vi "SA Initialize - TOI.vi"(8 "error in":errorcluster, 11 "RFmx Settings":T1 {"Attenuation"."Attenuation"."s2p File"."RFmx S-Parameters Orientation" items=["Port1 Towards DUT"=24000, "Port2 Towards DUT"=24001]; "Attenuation"."Attenuation"."Constant Attenuation"."RFmx External Attenuation (dB)" format="%.2f"; "Reference Level (dBm)" format="%.2f"}) -> (0 "error out":errorcluster, 3 "RFmx Session":refnum<k21>)   [LabVIEW 2023]
uses:
  Controls/RFmx Config - TOI.ctl
  FPT Shared VIs/De-embedding/RFmx Config.ctl
  <vilib>/RFmx/SpecAn/mx/RFmxSpecAn.llb/RFmxSpecAn Select Measurement (Single).vi
  <resource>/objmgr/RFmxSpecAn.rc
  <resource>/objmgr/RFmxInstr.rc
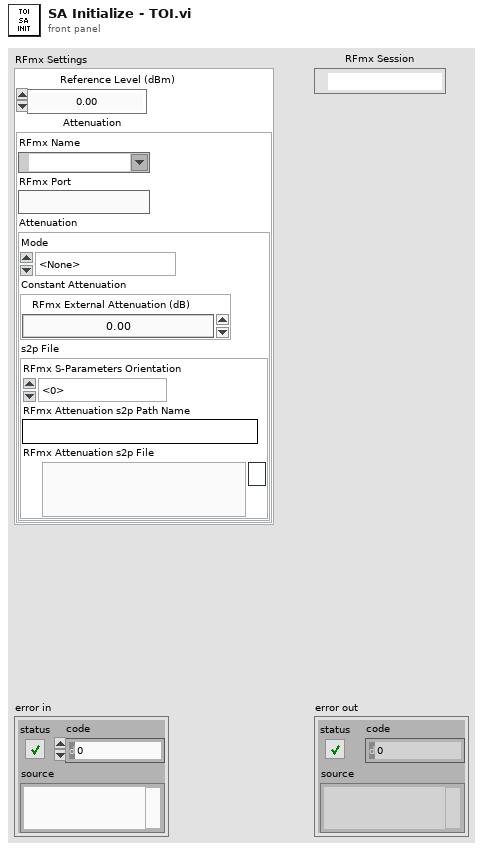
[diagram p1: front panel]
types:
  T1 = typedef "RFmx Config - TOI.ctl" = cluster{"Reference Level (dBm)":dbl, "Attenuation":T2}
  T2 = typedef "RFmx Config.ctl" = cluster{"RFmx Name":refnum<k15>, "RFmx Port":string, "Attenuation":cluster{"Mode":enum32{"<None>", "Constant Attenuation", "s2p File"}, "Constant Attenuation":cluster{"RFmx External Attenuation (dB)":dbl}, "s2p File":cluster{"RFmx S-Parameters Orientation":i32, "RFmx Attenuation s2p Path Name":string, "RFmx Attenuation s2p File":path}}}
  T3 = enum16{"ACP", "CCDF", "CHP", "FCnt", "Harmonics", "OBW", "SEM", "Spectrum", "Spur", "TXP", "AMPM", "DPD", "IQ", "IM", "NF", "PhaseNoise", "PAVT", "IDPD"}
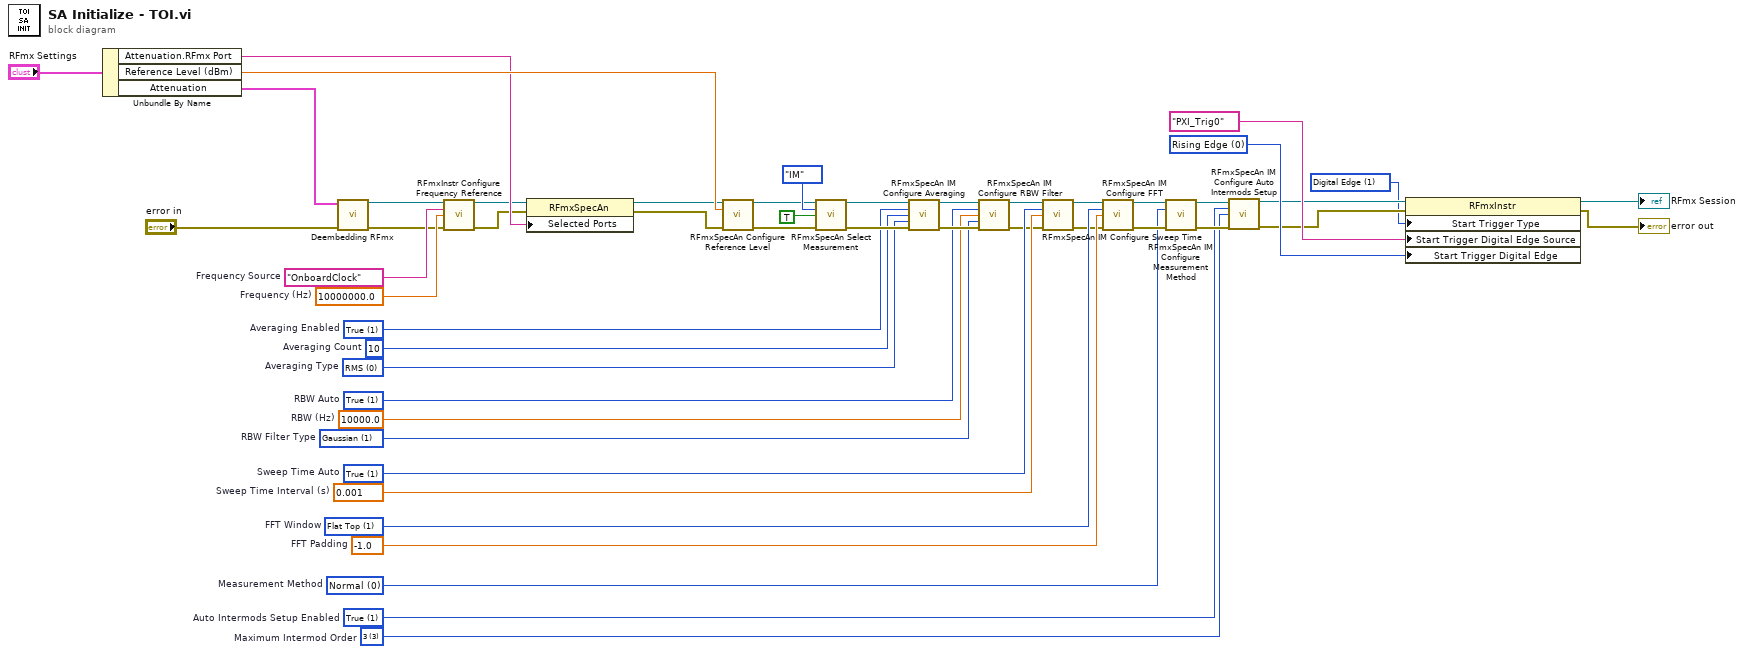
[diagram p0: block diagram]
diagram:
  w6 = 1 items=["None"=0, "Digital Edge"=1, "Software"=3] ("Start Trigger Type")
  w15 = 0 items=["Rising Edge", "Falling Edge"] ("Digital Edge")
  w39 = -1.0  # FFT Padding
  w38 = 1 items=["None", "Flat Top", "Hanning", "Hamming", "Gaussian", "Blackman", "Blackman-Harris", "Kaiser-Bessel"]  # FFT Window
  w29 = 0 items=["Normal", "Dynamic Range", "Segmented"]  # Measurement Method
  w22 = 1 items=["False", "True"]  # RBW Auto
  w23 = 10000.0  # RBW (Hz)
  w24 = 1 items=["FFT Based", "Gaussian", "Flat"]  # RBW Filter Type
  w26 = 0.001  # Sweep Time Interval (s)
  w25 = 1 items=["False", "True"]  # Sweep Time Auto
  w31 = 0 items=["RMS", "Log", "Scalar", "Max", "Min"]  # Averaging Type
  w21 = 10  # Averaging Count
  w30 = 1 items=["False", "True"]  # Averaging Enabled
  w18 = 10000000.0  # Frequency (Hz)
  w17 = "OnboardClock"  # Frequency Source
  w43 = 3 items=["3"=3, "5"=5, "7"=7, "9"=9]  # Maximum Intermod Order
  w42 = 1 items=["False", "True"]  # Auto Intermods Setup Enabled
  n1 = Unbundle By Name("RFmx Settings") -> ("Attenuation.RFmx Port"=w46:string, "Reference Level (dBm)"=w47:dbl, "Attenuation"=w1:T2)
  n2 = call "Deembedding RFmx.vi"("error in"="error in", "RFmx Settings"=w1) -> ("error out"=w4:errorcluster, "Refnum out"=w3:refnum<k21>)  [unwired: 8 in]
  n3 = call <vilib>:"RFmxInstr Configure Frequency Reference.vi"("Instrument Handle In"=w3, "Frequency Reference Source"=w17, "Frequency (Hz)"=w18, "error in (no error)"=w4) -> ("Instrument Handle Out"=w44:refnum<k21>, "error out"=w45:errorcluster)  [unwired: 10 in]
  n4 = property class="RFmxSpecAn"(reference=w44, error in=w45, "Selected Ports"=w46) -> (reference out=w10:refnum<k21>, error out=w9:errorcluster)
  n5 = call <vilib>:"RFmxSpecAn Configure Reference Level.vi"("Instrument Handle In"=w10, "Reference Level"=w47, "error in (no error)"=w9) -> ("Instrument Handle Out"=w8:refnum<k21>, "error out"=w5:errorcluster)  [unwired: 11 in]
  n6 = call-poly <vilib>:"RFmxSpecAn Select Measurement.vi"("Instrument Handle In"=w8, "Measurement"=T3."IM", "Enable All Traces"=TRUE, "error in (no error)"=w5) -> ("Instrument Handle Out"=w36:refnum<k21>, "error out"=w37:errorcluster)  [unwired: 10 in]
  n7 = call <vilib>:"RFmxSpecAn IM Configure Averaging.vi"("Instrument Handle In"=w36, "Averaging Enabled"=w30, "Averaging Count"=w21, "Averaging Type"=w31, "error in (no error)"=w37) -> ("Instrument Handle Out"=w32:refnum<k21>, "error out"=w33:errorcluster)  [unwired: 9 in]
  n8 = call <vilib>:"RFmxSpecAn IM Configure RBW Filter.vi"("Instrument Handle In"=w32, "RBW Auto"=w22, "RBW (Hz)"=w23, "RBW Filter Type"=w24, "error in (no error)"=w33) -> ("Instrument Handle Out"=w19:refnum<k21>, "error out"=w20:errorcluster)  [unwired: 9 in]
  n9 = call <vilib>:"RFmxSpecAn IM Configure Sweep Time.vi"("Instrument Handle In"=w19, "Sweep Time Auto"=w25, "Sweep Time Interval (s)"=w26, "error in (no error)"=w20) -> ("Instrument Handle Out"=w34:refnum<k21>, "error out"=w35:errorcluster)  [unwired: 10 in]
  n10 = call <vilib>:"RFmxSpecAn IM Configure FFT.vi"("Instrument Handle In"=w34, "FFT Window"=w38, "FFT Padding"=w39, "error in (no error)"=w35) -> ("Instrument Handle Out"=w40:refnum<k21>, "error out"=w41:errorcluster)  [unwired: 10 in]
  n11 = call <vilib>:"RFmxSpecAn IM Configure Measurement Method.vi"("Instrument Handle In"=w40, "Measurement Method"=w29, "error in (no error)"=w41) -> ("Instrument Handle Out"=w48:refnum<k21>, "error out"=w49:errorcluster)  [unwired: 11 in]
  n12 = call <vilib>:"RFmxSpecAn IM Configure Auto Intermods Setup.vi"("Instrument Handle In"=w48, "Auto Intermods Setup Enabled"=w42, "Maximum Intermod Order"=w43, "error in (no error)"=w49) -> ("Instrument Handle Out"=w14:refnum<k21>, "error out"=w13:errorcluster)  [unwired: 10 in]
  n13 = property class="RFmxInstr"(reference=w14, error in=w13, "Start Trigger Type"=w6, "Start Trigger Digital Edge Source"="PXI_Trig0" ("Digital Edge Source"), "Start Trigger Digital Edge"=w15) -> (reference out=→"RFmx Session":refnum<k21>, error out=→"error out":errorcluster)
